vi "transition.vi"(8 "error in (no error)":errorcluster, 10 "ContextData In":refnum<class "ContextData.lvclass">, 11 "User State 2 in":refnum<class "User State 2.lvclass">) -> (0 "error out":errorcluster, 2 "ContextData Out":refnum<class "ContextData.lvclass">, 3 "Next State":refnum<class "State.lvclass">)   [LabVIEW 2019, in "User State 2.lvclass"]
uses:
  User State 2.lvclass
  State/State.lvclass
  ContextData/ContextData.lvclass
  Wait Event/Wait Event.lvclass
  C:/Users/Felipe-PC/Documents/Projetos/Projetos Github/OOP-State-Machine/State/State.lvclass
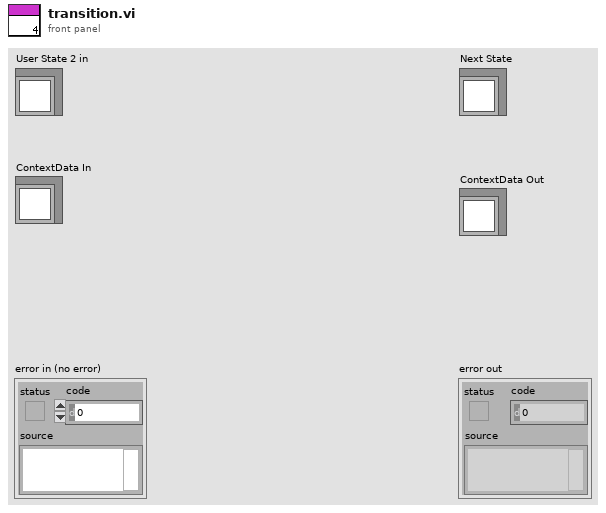
[diagram p1: front panel]
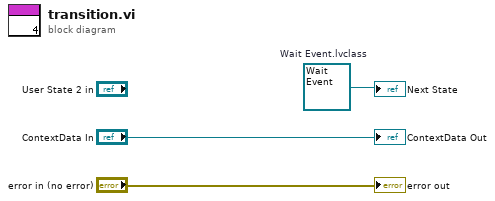
[diagram p0: block diagram]
diagram:
  w1 = refnum<class "Wait Event.lvclass"> refnum  # Wait Event.lvclass
  "error out" <- "error in (no error)"
  "Next State" <- w1
  "ContextData Out" <- "ContextData In"
